vi "Pre Launch Init.vi"(11 "Timing Engine in":refnum<class "Timing Engine.lvclass">) -> (0 "error out":errorcluster, 3 "Timing Engine out":refnum<class "Timing Engine.lvclass">)   [LabVIEW 2016, in "Assert API Components.lvlib" / "Assert Display.lvlib" / "Timing Engine.lvlib" / "Timing Engine.lvclass"]
doc: "(<B>Filename</B>: Actor Framework.lvlib:Actor.lvclass:Pre Launch Init.vi)\n\nDefines behavior that occurs after the Launch Nested Actor method is invoked but before the actor's Actor Core method begins running.\n\nBy default, this method does nothing. A descendant class may override it to define behavior."
uses:
  Timing Engine.lvclass
  Timing Engine.lvclass/Timing Engine.ctl
  Base UI Actor/Base UI Actor/Base UI Actor.lvclass
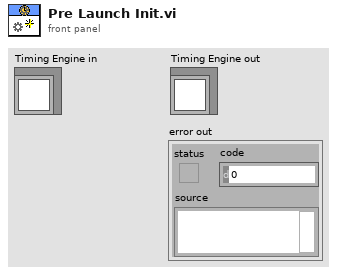
[diagram p1: front panel]
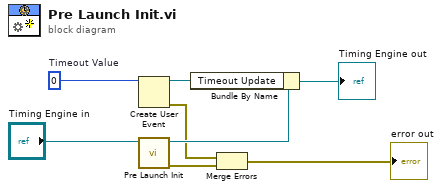
[diagram p0: block diagram]
diagram:
  w5 = 0  # Timeout Value
  n1 = Create User Event(user event datatype=w5) -> (user event=w3:refnum<user-event>, error out=w1:errorcluster)  [unwired: 1 in]
  n2 = call-parent "Pre Launch Init.vi"("Base UI Actor in"="Timing Engine in") -> ("error out"=w8:errorcluster, "Base UI Actor out"=w7:refnum<class "Timing Engine.lvclass">)  [unwired: 9 in]
  n3 = Bundle By Name(cluster=w7, "Timeout Update"=w3) -> (→"Timing Engine out":refnum<class "Timing Engine.lvclass">)
  n4 = Merge Errors(w1, w8) -> (→"error out":errorcluster)
